vi "Global Var.vi"() -> ()   [LabVIEW 2014]
panel:
  in  "header":dbl
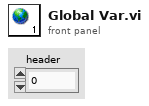
[diagram p1: front panel]
diagram:
